vi "a.vi"() -> ()   [LabVIEW 2012]
uses:
  <vilib>/Analysis/NI_AALPro.lvlib
  <vilib>/Analysis/2dsp.llb/Real FFT.vi
  <vilib>/DAQmx/read.llb/DAQmx Read (Analog 2D DBL NChan NSamp).vi
panel:
  in  "Arean på solcellen":dbl(slide) scale=0.0..10.0
  in  "Resistansen storlek":dbl
  in  "Casenummer":dbl
  out "XY Graph 2":cluster{"Y":dbl[], "Y":dbl[]}[](graph)
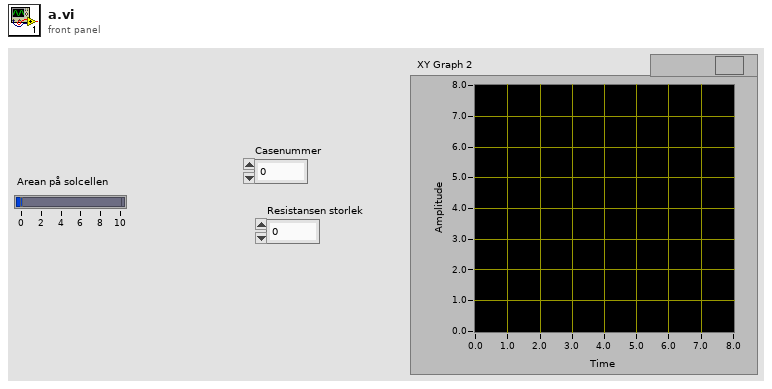
[diagram p1: front panel]
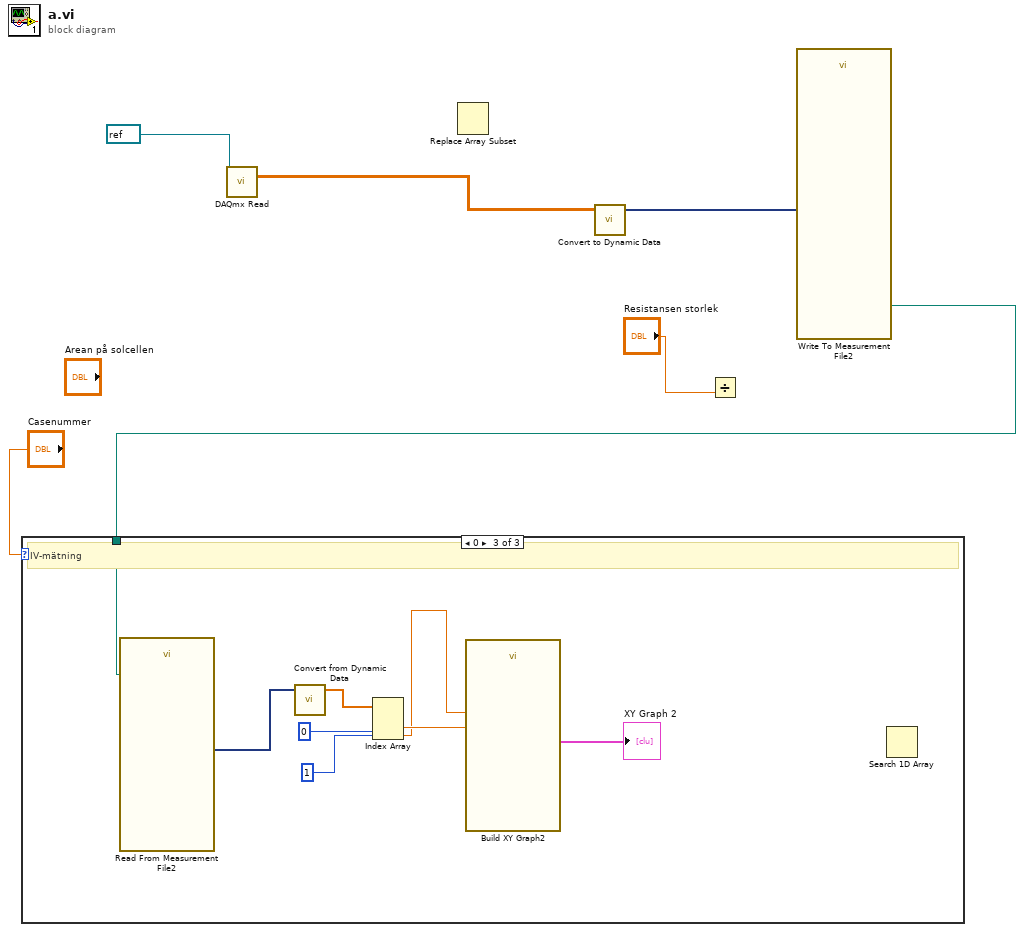
[diagram p0: block diagram]
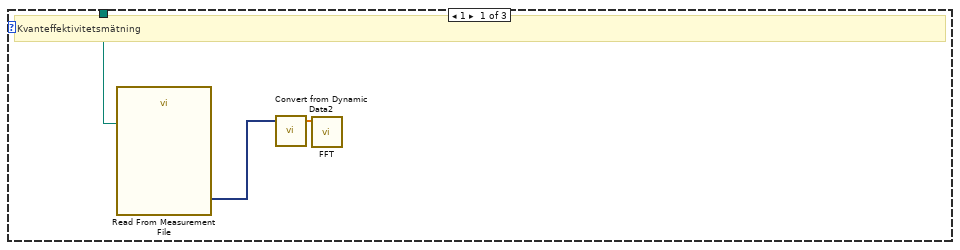
[diagram p2: hidden frame]
diagram:
  n1 = call-poly <vilib>:"DAQmx Read.vi"("task/channels in"=refnum<k21> refnum) -> ("data"=w2:dbl[][])  [unwired: 12 in, 2 out]
  n2 = Replace Array Subset() -> ()  [unwired: 3 in, 1 out]
  n3 = call "Convert to Dynamic Data"("2D Array"=w2) -> ("Dynamic Data Type"=w1:dynamicdata)  [unwired: 3 in]
  n4 = Divide(y="Resistansen storlek") -> ()  [unwired: 1 in, 1 out]
  n5 = call "Write To Measurement File2"("Signals"=w1) -> ("Filename Out"=w5:path)  [unwired: 16 in, 2 out]
  n6 = case shown="0" "Casenummer" {
    tunnel: w5 -> [w9 _ w10]
    frame 1 {
      # "Kvanteffektivitetsmätning"
      n7 = call "Read From Measurement File"("Filename"=w9) -> ("Signals"=w8:dynamicdata)  [unwired: 5 in, 5 out]
      n8 = call "Convert from Dynamic Data2"("Dynamic Data Type"=w8) -> ("Array"=w7:dbl[])  [unwired: 3 in]
      n9 = call-poly <vilib>:"FFT.vi"("X"=w7) -> ()  [unwired: 9 in, 2 out]
    }
    frame 2 {
      # "Kromatisk frekvensstyrning"
    }
    frame 0 {
      # "IV-mätning"
      n10 = call "Read From Measurement File2"("Filename"=w10) -> ("Signals"=w16:dynamicdata)  [unwired: 5 in, 5 out]
      n11 = call "Convert from Dynamic Data"("Dynamic Data Type"=w16) -> ("Array"=w15:dbl[])  [unwired: 3 in]
      n12 = Index Array(array=w15, index #1=0 ("index"), index #3=1 ("index")) -> (element #2=w12:dbl, element #3=w11:dbl)  [unwired: 1 in, 1 out]
      n13 = call "Build XY Graph2"("Y Input"=w12, "X Input"=w11) -> ("XY Graph"=→"XY Graph 2":cluster{"Y":dbl[], "Y":dbl[]}[])  [unwired: 3 in, 6 out]
      n14 = Search 1D Array() -> ()  [unwired: 3 in, 1 out]
    }
  }
